vi "Barcode-Indentify-Set_Api.vi"(8 "Error In":errorcluster, 11 "Session In":T2) -> (0 "Error Out":errorcluster, 3 "Progressing Data":T3)   [LabVIEW 2019]
uses:
  <vilib>/userDefined/High Color/IMAQdx.ctl
  <vilib>/vision/Image Controls.llb/IMAQ Image.ctl
  <vilib>/vision/driver/NI_Vision_Acquisition_Software.lvlib
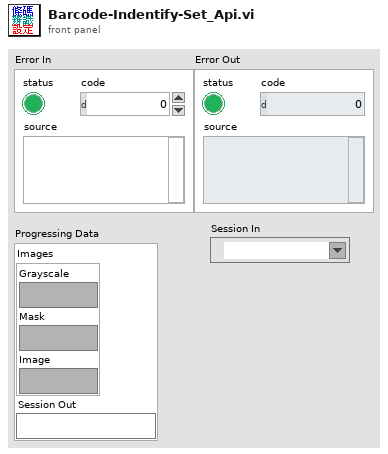
[diagram p1: front panel]
types:
  T1 = typedef "IMAQ Image.ctl" = refnum<image>
  T2 = typedef "IMAQdx.ctl" = refnum<k21>
  T3 = cluster{"Images":cluster{"Grayscale":T1, "Mask":T1, "Image":T1}, "Session Out":T2}
  T4 = cluster{"Images":cluster{"Image":T1, "Mask":T1, "Grayscale":T1}, "Session Out":T2}
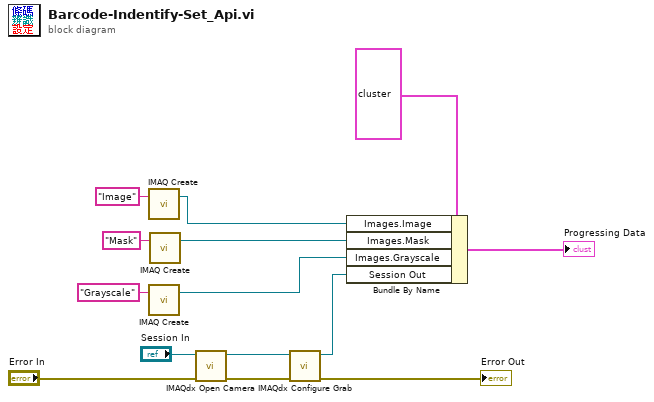
[diagram p0: block diagram]
diagram:
  n1 = call "IMAQ Create"("Image Name"="Image") -> ("New Image"=w3:T1)  [unwired: 4 in, 1 out]
  n2 = call "IMAQ Create"("Image Name"="Grayscale") -> ("New Image"=w5:T1)  [unwired: 4 in, 1 out]
  n3 = call "IMAQ Create"("Image Name"="Mask") -> ("New Image"=w4:T1)  [unwired: 4 in, 1 out]
  n4 = call <vilib>:"IMAQdx Open Camera.vi"("error in"="Error In", "Session In"="Session In") -> ("error out"=w12:errorcluster, "Session Out"=w11:T2)  [unwired: 8 in]
  n5 = call <vilib>:"IMAQdx Configure Grab.vi"("error in"=w12, "Session In"=w11) -> ("error out"=→"Error Out":errorcluster, "Session Out"=w6:T2)  [unwired: 8 in]
  n6 = Bundle By Name(cluster=T4 {"Images"={"Image"=refnum, "Mask"=refnum, "Grayscale"=refnum}, "Session Out"=""} ("Progressing Data 2"), "Images.Image"=w3, "Images.Mask"=w4, "Images.Grayscale"=w5, "Session Out"=w6) -> (→"Progressing Data":T4)
